vi "AO SCTR Messenger.vi"(0 "Notifier Name":string, 2 "Actions":T1, 5 "Offset (V)":dbl=-1.0, 7 "Amplitude (V)":dbl=-1.0, 9 "Samples Per Channel":i32=-1, 11 "Start Delay (ms)":dbl=-1.0, 13 "Exposure Time (s)":dbl=-1.0) -> (4 "Notifier Name (Dup)":string)   [LabVIEW 2020]
uses:
  AO SCTR Type Defs/AO SCTR Actions.ctl
  AO SCTR Type Defs/AO SCTR Notifier Type.ctl
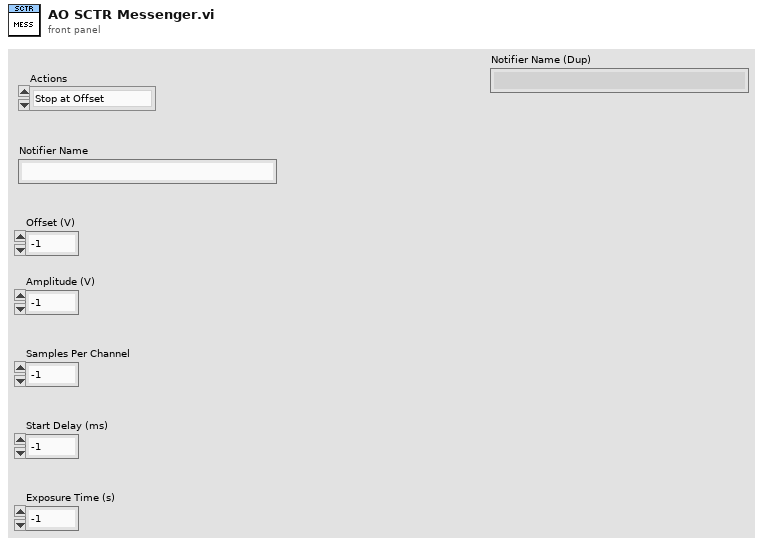
[diagram p1: front panel]
types:
  T1 = typedef "AO SCTR Actions.ctl" = enum16{"Stop at Offset", "Update and Run", "Quit"}
  T2 = typedef "AO SCTR Notifier Type.ctl" = cluster{"Actions":T1, "Offset (V)":dbl, "Amplititude (V)":dbl, "Samples Per Channel":i32, "Start Delay (ms)":dbl, "Running?":bool, "Exposure Time (s)":dbl}
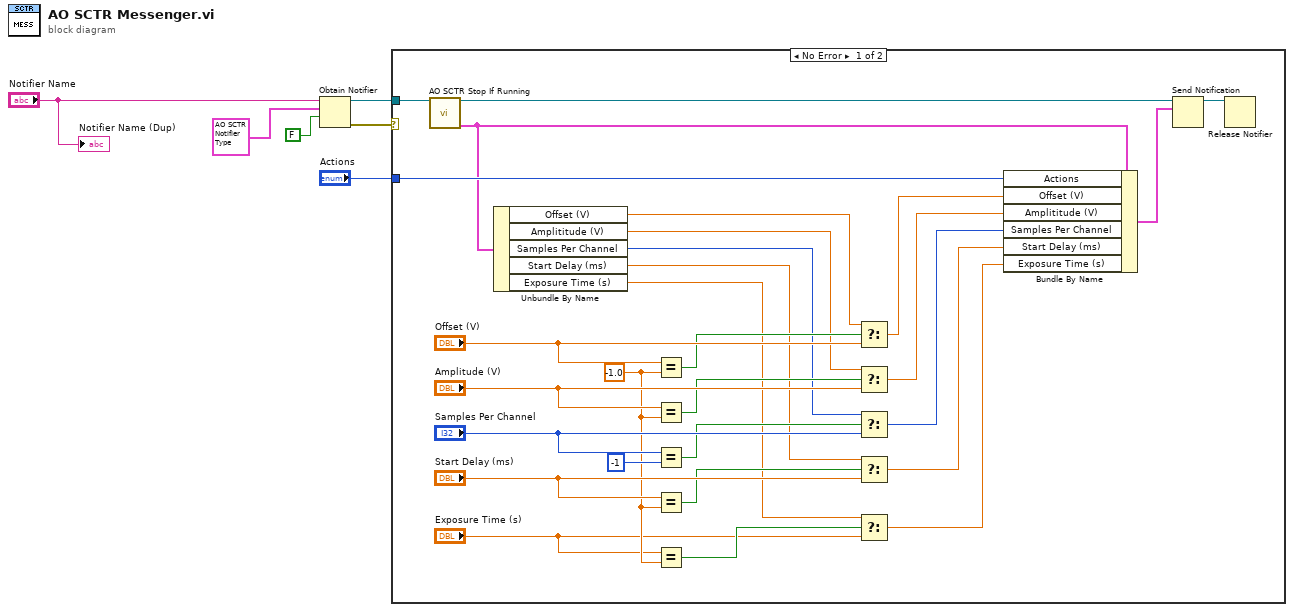
[diagram p0: block diagram]
diagram:
  n1 = Obtain Notifier(name (unnamed)="Notifier Name", notification data type=T2 {"Actions"=enum."Stop at Offset", "Offset (V)"=0.0, "Amplititude (V)"=0.0, "Samples Per Channel"=0, "Start Delay (ms)"=0.0, "Running?"=FALSE, "Exposure Time (s)"=0.0} ("Waveform Settings 2"), create if not found? (T)=FALSE) -> (notifier out=w2:refnum<notifier>, error out=w3:errorcluster)  [unwired: 1 in, 1 out]
  n2 = case shown="No Error" w3 {
    tunnel: w2 -> [w34 _]
    tunnel: "Actions" -> [w33 _]
    frame No Error {
      w11 = -1.0 ("y")
      n3 = call "AO SCTR Stop If Running.vi"("AO SCTR Notifier"=w34) -> ("AO SCTR Notifier (Dup)"=w31:refnum<notifier>, "Latest Notification"=w12:T2)  [unwired: 13 in]
      n4 = Unbundle By Name(w12) -> ("Offset (V)"=w20:dbl, "Amplititude (V)"=w19:dbl, "Samples Per Channel"=w18:i32, "Start Delay (ms)"=w17:dbl, "Exposure Time (s)"=w9:dbl)
      n5 = Equal?(x="Offset (V)", y=w11) -> (x = y?=w24:bool)
      n6 = Equal?(x="Amplitude (V)", y=w11) -> (x = y?=w23:bool)
      n7 = Equal?(x="Samples Per Channel", y=-1) -> (x = y?=w22:bool)
      n8 = Equal?(x="Start Delay (ms)", y=w11) -> (x = y?=w21:bool)
      n9 = Equal?(x="Exposure Time (s)", y=w11) -> (x = y?=w10:bool)
      n10 = Select(t=w20, s=w24, f="Offset (V)") -> (s? t:f=w16:dbl)
      n11 = Select(t=w19, s=w23, f="Amplitude (V)") -> (s? t:f=w15:dbl)
      n12 = Select(t=w18, s=w22, f="Samples Per Channel") -> (s? t:f=w14:i32)
      n13 = Select(t=w17, s=w21, f="Start Delay (ms)") -> (s? t:f=w13:dbl)
      n14 = Select(t=w9, s=w10, f="Exposure Time (s)") -> (s? t:f=w7:dbl)
      n15 = Bundle By Name(cluster=w12, "Actions"=w33, "Offset (V)"=w16, "Amplititude (V)"=w15, "Samples Per Channel"=w14, "Start Delay (ms)"=w13, "Exposure Time (s)"=w7) -> (w30:T2)
      n16 = Send Notification(notification=w30, notifier=w31) -> (notifier out=w32:refnum<notifier>)  [unwired: 1 in, 1 out]
      n17 = Release Notifier(notifier=w32) -> ()  [unwired: 2 in, 3 out]
    }
    frame Error {
    }
  }
  "Notifier Name (Dup)" <- "Notifier Name"
